vi "Get Temperature.vi"(8 "error in":errorcluster, 11 "PPT in":refnum<class "PPT.lvclass">) -> (0 "error out":errorcluster, 2 "T":dbl, 3 "PPT out":refnum<class "PPT.lvclass">)   [LabVIEW 2014, in "PPT.lvclass"]
uses:
  PPT.lvclass
  PPT.lvclass/PPT.ctl
  Reusable/Session APIs/Serial/Public/Get Data/Get String.vi
  Reusable/Session APIs/Text Communication/Text Device Session.lvclass
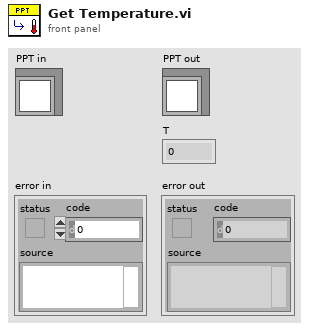
[diagram p1: front panel]
types:
  T1 = typedef "Session - Root.lvclass/Session Handle.ctl" = refnum<data-value>
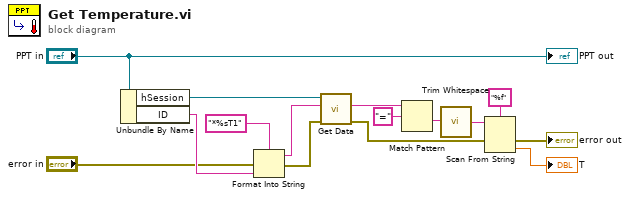
[diagram p0: block diagram]
diagram:
  n1 = Unbundle By Name("PPT in") -> ("hSession"=w13:T1, "ID"=w11:string)
  n2 = Format Into String(format string="*%sT1", error in="error in", w11) -> (resulting string=w10:string, error out=w4:errorcluster)  [unwired: 1 in]
  n3 = call-poly "Get Data.vi"("error in"=w4, "CMD"=w10, "handle in"=w13) -> ("error out"=w3:errorcluster, "DataOut"=w9:string)  [unwired: 6 in, 1 out]
  n4 = Match Pattern(string=w9, regular expression="=") -> (after substring=w7:string)  [unwired: 1 in, 3 out]
  n5 = call <vilib>:"Trim Whitespace.vi"("string"=w7) -> ("trimmed string"=w6:string)  [unwired: 1 in]
  n6 = Scan From String(format string="%f", input string=w6, error in=w3) -> (error out=→"error out":errorcluster, output 1=→"T":dbl)  [unwired: 2 in, 2 out]
  "PPT out" <- "PPT in"
